vi "Moving Ripple-Create.vi"(0 "Moving Ripple":T1, 5 "Sampling Rate (Hz)":dbl, 7 "Npts":i32) -> (4 "Data":T3, 6 "Array":dbl[](array[numeric]), 15 "error out":errorcluster)   [LabVIEW 2020]
uses:
  Moving Ripple.Data.ctl
  Moving Ripple.ctl
  Moving Ripple.Params.ctl
  Utility VIs/Math VIs/LinSpace (x0-dx-npts).vi
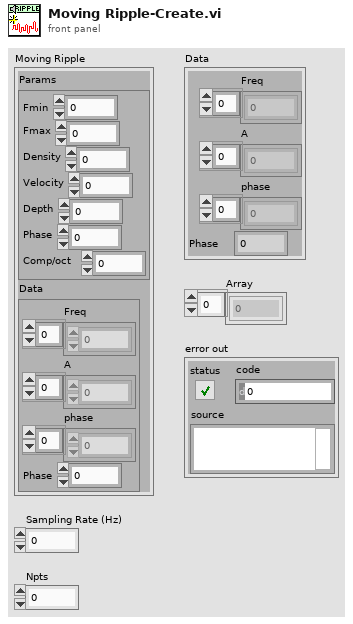
[diagram p1: front panel]
types:
  T1 = typedef "Moving Ripple.ctl" = cluster{"Params":T2, "Data":T3}
  T2 = typedef "Moving Ripple.Params.ctl" = cluster{"Fmin":dbl, "Fmax":dbl, "Density":dbl, "Velocity":dbl, "Depth":dbl, "Phase":dbl, "Comp/oct":i32}
  T3 = typedef "Moving Ripple.Data.ctl" = cluster{"Freq":dbl[], "A":dbl[], "phase":dbl[], "Phase":dbl}
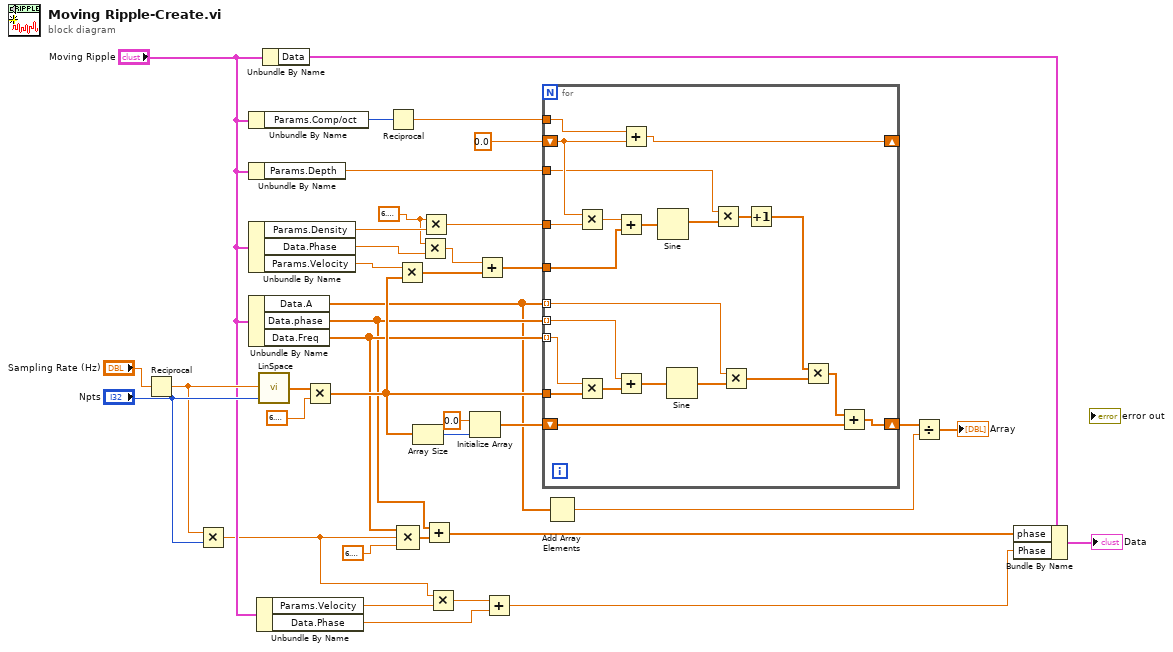
[diagram p0: block diagram]
diagram:
  w32 = 6.283185307179586
  n1 = Reciprocal(x="Sampling Rate (Hz)") -> (1/x=w17:dbl)
  n2 = Multiply(x=w17, y="Npts") -> (x*y=w7:dbl)
  n3 = Unbundle By Name("Moving Ripple") -> ("Params.Comp/oct"=w24:i32)
  n4 = Unbundle By Name("Moving Ripple") -> ("Params.Depth"=w22:dbl)
  n5 = Unbundle By Name("Moving Ripple") -> ("Params.Density"=w34:dbl, "Data.Phase"=w33:dbl, "Params.Velocity"=w35:dbl)
  n6 = Unbundle By Name("Moving Ripple") -> ("Data.A"=w2:dbl[], "Data.phase"=w10:dbl[], "Data.Freq"=w16:dbl[])
  n7 = Unbundle By Name("Moving Ripple") -> ("Params.Velocity"=w8:dbl, "Data.Phase"=w5:dbl)
  n8 = call-poly "LinSpace.vi"("npts"="Npts", "dx"=w17) -> ("Array"=w37:dbl[])  [unwired: 2 in, 1 out]
  n9 = Unbundle By Name("Moving Ripple") -> ("Data"=w14:T3)
  n10 = Multiply(x=w37, y=6.283185307179586) -> (x*y=w21:dbl[])
  n11 = Reciprocal(x=w24) -> (1/x=w23:dbl)
  n12 = Multiply(x=w35, y=w21) -> (x*y=w27:dbl[])
  n13 = Compound Arithmetic op=MULTIPLY(w16, w7, 6.283185307179586) -> (w12:dbl[])
  n14 = Array Size(array=w21) -> (size(s)=w31:i32)
  n15 = Multiply(x=w32, y=w33) -> (x*y=w25:dbl)
  n16 = Multiply(x=w32, y=w34) -> (x*y=w29:dbl)
  n17 = Add(x=w10, y=w12) -> (x+y=w11:dbl[])
  n18 = Multiply(x=w7, y=w8) -> (x*y=w6:dbl)
  n19 = Initialize Array(0.0 ("element"), w31) -> (w20:dbl[])
  n20 = Add(x=w25, y=w27) -> (x+y=w26:dbl[])
  n21 = Add(x=w6, y=w5) -> (x+y=w4:dbl)
  n22 = for {
    tunnel: w2 -> [w39] mode=indexing
    tunnel: w29 -> [w60]
    shift-right: [w54] -> _
    shift-left: 0.0 -> [w56]
    tunnel: w26 -> [w58]
    tunnel: w23 -> [w55]
    tunnel: w22 -> [w52]
    tunnel: w21 -> [w50]
    tunnel: w10 -> [w47] mode=indexing
    tunnel: w16 -> [w49] mode=indexing
    shift-right: [w40] -> w19
    shift-left: w20 -> [w42]
    n23 = Multiply(x=w56, y=w60) -> (x*y=w59:dbl)
    n24 = Multiply(x=w49, y=w50) -> (x*y=w48:dbl[])
    n25 = Add(x=w59, y=w58) -> (x+y=w57:dbl[])
    n26 = Add(x=w47, y=w48) -> (x+y=w46:dbl[])
    n27 = Add(x=w55, y=w56) -> (x+y=w54:dbl)
    n28 = Sine(x=w57) -> (sin(x)=w53:dbl[])
    n29 = Sine(x=w46) -> (sin(x)=w45:dbl[])
    n30 = Multiply(x=w52, y=w53) -> (x*y=w51:dbl[])
    n31 = Multiply(x=w39, y=w45) -> (x*y=w44:dbl[])
    n32 = Increment(x=w51) -> (x+1=w43:dbl[])
    n33 = Multiply(x=w43, y=w44) -> (x*y=w41:dbl[])
    n34 = Add(x=w41, y=w42) -> (x+y=w40:dbl[])
  }
  n35 = Add Array Elements(numeric array=w2) -> (sum=w1:dbl)
  n36 = Divide(x=w19, y=w1) -> (x/y=→"Array":dbl[])
  n37 = Bundle By Name(cluster=w14, "phase"=w11, "Phase"=w4) -> (→"Data":T3)
